vi "Voltage Sweep.vi"() -> ()   [LabVIEW 2012]
doc: "This example demonstrates how to continuously re-generate analog output data from a buffer in your computer's memory.\n\nRefer to your device documentation for pinouts and hardware capabilities."
uses:
  <vilib>/DAQmx/write.llb/DAQmx Write (Analog 1D DBL 1Chan NSamp).vi
  <vilib>/DAQmx/create/channels.llb/DAQmx Create Channel (AO-Voltage-Basic).vi
  <vilib>/DAQmx/configure/timing.llb/DAQmx Timing (Sample Clock).vi
  <vilib>/DAQmx/configure/trigger.llb/DAQmx Start Trigger (Digital Edge).vi
  <vilib>/DAQmx/configure/trigger.llb/DAQmx Start Trigger (Analog Edge).vi
  <vilib>/DAQmx/miscellaneous.llb/DAQmx Fill In Error Info.vi
  <resource>/objmgr/daqmx.rc
panel:
  in  "Step Size":dbl=0.01
  in  "Ending Voltage":dbl=10.0
  in  "Starting Voltage":dbl=6.0
  in  "Trigger Type":T1(tab)
  in  "Edge":i32(ring)=10280 items=["Rising"=10280, "Falling"=10171]
  in  "Digital Trigger Source":tag
  in  "Level (V)":dbl format="%0.2f"
  in  "Hysteresis (V)":dbl
  in  "Slope":i32(ring)=10280 items=["Rising"=10280, "Falling"=10171]
  in  "Analog Trigger Source":string="APFI0"
  in  "Pause When":i32(ring)=10192 items=["High"=10192, "Low"=10214]
  in  "Pause Trigger Source":tag
  in  "Stop":bool
  in  "Sample Rate":dbl=1.0
  in  "Sample Clock Source":tag="OnboardClock"
  in  "Max Voltage":dbl=10.0
  in  "Min Voltage":dbl
  in  "Physical Channel(s)":tag="Dev1/ao0"
  # "Channel Settings"
  # "Timing and Buffer Settings"
  # "Trigger Settings"
  # "To configure and use a start trigger you must have the necessary tab selected above.  Not all hardware supports triggering--refer to your device documentation for more info."
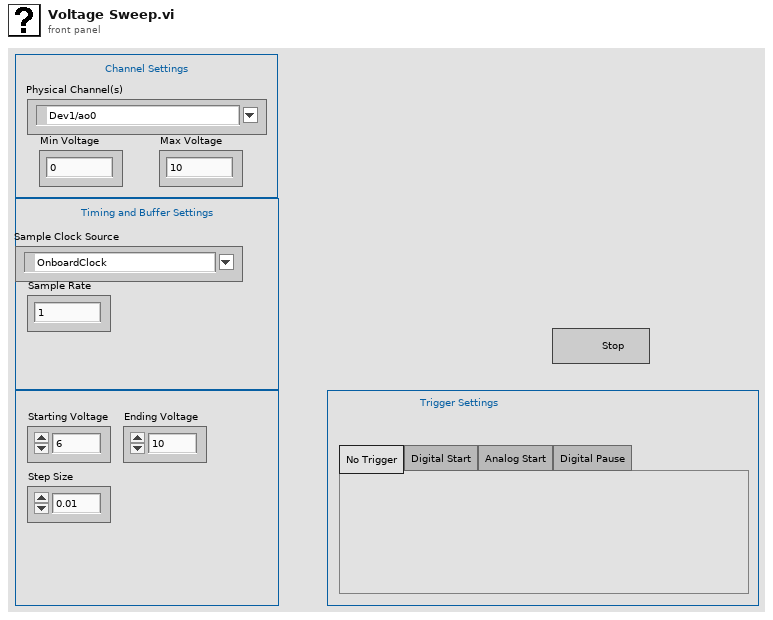
[diagram p1: front panel]
types:
  T1 = enum32{"No Trigger", "Digital Start", "Analog Start", "Digital Pause"}
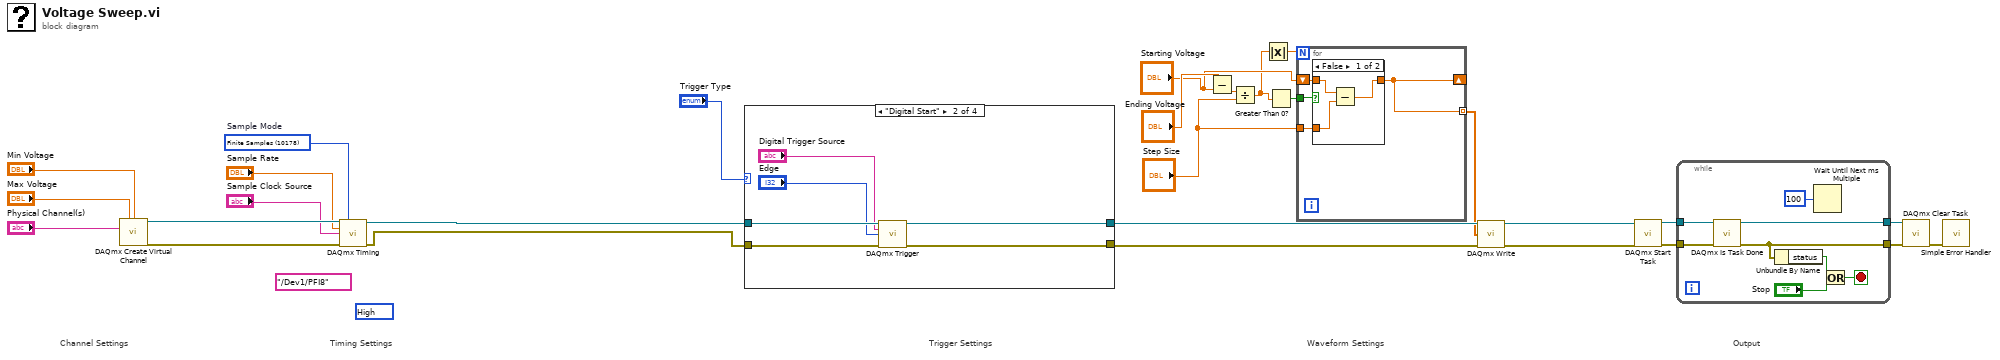
[diagram p0: block diagram]
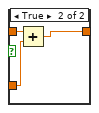
[diagram p2: hidden frame]
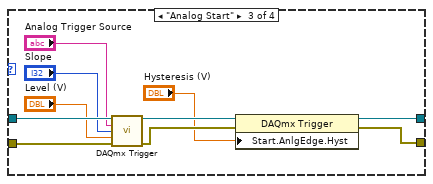
[diagram p4: hidden frame]
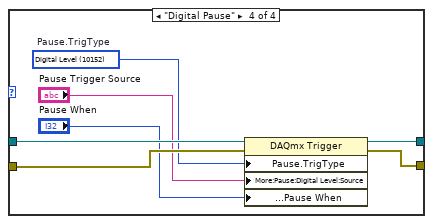
[diagram p5: hidden frame]
diagram:
  (unwired) 10192 items=["High"=10192, "Low"=10214] ("Pause.DigLvl.When")
  (unwired) tag "/Dev1/PFI8" ("Pause.DigLvl.Src")
  w28 = 10178 items=["Finite Samples"=10178, "Continuous Samples"=10123, "Hardware Timed Single Point"=12522]  # Sample Mode
  # "Output"
  # "Trigger Settings"
  # "Waveform Settings"
  # "Timing Settings"
  # "Channel Settings"
  n1 = call-poly <vilib>:"DAQmx Create Virtual Channel.vi"("maximum value"="Max Voltage", "minimum value"="Min Voltage", "physical channels"="Physical Channel(s)") -> ("task out"=w26:refnum<k21>, "error out"=w27:errorcluster)  [unwired: 11 in]
  n2 = call-poly <vilib>:"DAQmx Timing.vi"("task/channels in"=w26, "sample mode"=w28, "rate"="Sample Rate", "source"="Sample Clock Source", "error in"=w27) -> ("task out"=w2:refnum<k21>, "error out"=w1:errorcluster)  [unwired: 9 in]
  n3 = case shown="\"Digital Start\"" "Trigger Type" {
    tunnel: w2 -> [w30 w36 w46 w53]
    tunnel: w1 -> [w29 w35 w45 w50]
    tunnel: [w30 w34 w43 w52] -> w13
    tunnel: [w29 w33 w42 w51] -> w12
    frame "No Trigger", Default {
    }
    frame "Digital Start" {
      n4 = call-poly <vilib>:"DAQmx Trigger.vi"("task/channels in"=w36, "source"="Digital Trigger Source", "edge"="Edge", "error in"=w35) -> ("task out"=w34:refnum<k21>, "error out"=w33:errorcluster)  [unwired: 10 in]
    }
    frame "Analog Start" {
      n5 = call-poly <vilib>:"DAQmx Trigger.vi"("task/channels in"=w46, "source"="Analog Trigger Source", "slope"="Slope", "level"="Level (V)", "error in"=w45) -> ("task out"=w41:refnum<k21>, "error out"=w40:errorcluster)  [unwired: 9 in]
      n6 = property class="DAQmx Trigger"(reference=w41, error in=w40, "Start.AnlgEdge.Hyst"="Hysteresis (V)") -> (reference out=w43:refnum<k21>, error out=w42:errorcluster)
    }
    frame "Digital Pause" {
      w49 = 10152 items=["Analog Level"=10101, "Analog Window"=10103, "Digital Level"=10152, "Digital Pattern"=10398, "None"=10230]  # Pause.TrigType
      n7 = property class="DAQmx Trigger"(reference=w53, error in=w50, "Pause.TrigType"=w49, "More:Pause:Digital Level:Source"="Pause Trigger Source", "More:Pause:Digital Level:Pause When"="Pause When") -> (reference out=w52:refnum<k21>, error out=w51:errorcluster)
    }
  }
  n8 = Subtract(x="Ending Voltage", y="Starting Voltage") -> (x-y=w11:dbl)
  n9 = Divide(x=w11, y="Step Size") -> (x/y=w3:dbl)
  n10 = Absolute Value(x=w3) -> (abs(x)=w5:dbl)
  n11 = Greater Than 0?(x=w3) -> (x > 0?=w4:bool)
  n12 = for {
    N: w5 -> [_]
    shift-right: [w55] -> _
    shift-left: "Starting Voltage" -> [w57]
    tunnel: "Step Size" -> [w56]
    tunnel: [w55] -> w7 mode=indexing
    tunnel: w4 -> [w54]
    n13 = case shown="False" w54 {
      tunnel: w57 -> [w60 w63]
      tunnel: w56 -> [w59 w62]
      tunnel: [w58 w61] -> w55
      frame False {
        n14 = Subtract(x=w60, y=w59) -> (x-y=w58:dbl)
      }
      frame True {
        n15 = Add(x=w63, y=w62) -> (x+y=w61:dbl)
      }
    }
  }
  n16 = call-poly <vilib>:"DAQmx Write.vi"("task/channels in"=w13, "data"=w7, "error in"=w12) -> ("task out"=w15:refnum<k21>, "error out"=w14:errorcluster)  [unwired: 10 in, 1 out]
  n17 = call <vilib>:"DAQmx Start Task.vi"("task/channels in"=w15, "error in"=w14) -> ("task out"=w25:refnum<k21>, "error out"=w24:errorcluster)  [unwired: 12 in]
  n18 = while {
    tunnel: w25 -> [w71]
    tunnel: w24 -> [w70]
    tunnel: [w67] -> w22
    tunnel: [w68] -> w23
    stop <- w69 stop-if-true
    n19 = call <vilib>:"DAQmx Is Task Done.vi"("task/channels in"=w71, "error in"=w70) -> ("task out"=w68:refnum<k21>, "error out"=w67:errorcluster)  [unwired: 11 in, 1 out]
    n20 = Unbundle By Name(w67) -> ("status"=w66:bool)
    n21 = Wait Until Next ms Multiple(millisecond multiple=u32 100) -> ()  [unwired: 1 out]
    n22 = Or(x=w66, y="Stop") -> (x .or. y?=w69:bool)
  }
  n23 = call <vilib>:"DAQmx Clear Task.vi"("task in"=w23, "error in"=w22) -> ("error out"=w21:errorcluster)  [unwired: 13 in]
  n24 = call <vilib>:"Simple Error Handler.vi"("error in (no error)"=w21) -> ()  [unwired: 4 in, 5 out]
